vi "Cairo.CloseConnectionFromFile.vi"(11 "RefNum":T1) -> (0 "Error Out":errorcluster)   [LabVIEW 2019]
uses:
  <vilib>/Utility/config.llb/Config Data RefNum.ctl
  <vilib>/Utility/config.llb/NI_LVConfig.lvlib
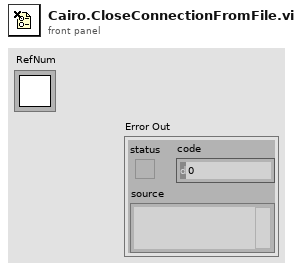
[diagram p1: front panel]
types:
  T1 = typedef "NI_LVConfig.lvlib/Config Data RefNum.ctl" = refnum<k1>
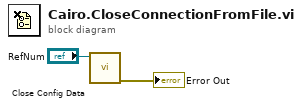
[diagram p0: block diagram]
diagram:
  n1 = call <vilib>:"Close Config Data.vi"("refnum"="RefNum") -> ("error out"=→"Error Out":errorcluster)  [unwired: 9 in, 1 out]
